vi "canDataSort.vi"() -> ()   [LabVIEW 2023] (continued)
"Min"=0.0, "Max"=65.535, "ScaleFac"=0.001, "ScaleOff"=0.0}, {"1FFFFFFC", "Frame"="PCINPUT\ndatabase", "NameShort"="PCRXMsg7", "StartBit"=48, "NumBits"=16, "Min"=0.0, "Max"=65.535, "ScaleFac"=0.001, "ScaleOff"=0.0}, {"1FFFFFFD", "Frame"="PCOUTPUT\ndatabase", "NameShort"="PCTXMsg1", "StartBit"=0, "NumBits"=16, "Min"=0.0, "Max"=65.535, "ScaleFac"=0.001, "ScaleOff"=0.0}, {"1FFFFFFD", "Frame"="PCOUTPUT\ndatabase", "NameShort"="PCTXMsg3", "StartBit"=16, "NumBits"=16, "Min"=0.0, "Max"=65.535, "ScaleFac"=0.001, "ScaleOff"=0.0}, {"1FFFFFFD", "Frame"="PCOUTPUT\ndatabase", "NameShort"="PCTXMsg5", "StartBit"=32, "NumBits"=16, "Min"=0.0, "Max"=65.535, "ScaleFac"=0.001, "ScaleOff"=0.0}, {"1FFFFFFD", "Frame"="PCOUTPUT\ndatabase", "NameShort"="PCTXMsg7", "StartBit"=48, "NumBits"=16, "Min"=0.0, "Max"=65.535, "ScaleFac"=0.001, "ScaleOff"=0.0}, {"1FFFFFFE", "Frame"="PCRX\ndatabase", "NameShort"="PCRXMsg1", "StartBit"=0, "NumBits"=8, "Min"=0.0, "Max"=255.0, "ScaleFac"=1.0, "ScaleOff"=0.0}, {"1FFFFFFE", "Frame"="PCRX\ndatabase", "NameShort"="PCRXMsg2", "StartBit"=8, "NumBits"=8, "Min"=0.0, "Max"=255.0, "ScaleFac"=1.0, "ScaleOff"=0.0}, {"1FFFFFFE", "Frame"="PCRX\ndatabase", "NameShort"="PCRXMsg3", "StartBit"=16, "NumBits"=8, "Min"=0.0, "Max"=255.0, "ScaleFac"=1.0, "ScaleOff"=0.0}, {"1FFFFFFE", "Frame"="PCRX\ndatabase", "NameShort"="PCRXMsg4", "StartBit"=24, "NumBits"=8, "Min"=0.0, "Max"=255.0, "ScaleFac"=1.0, "ScaleOff"=0.0}, {"1FFFFFFE", "Frame"="PCRX\ndatabase", "NameShort"="PCRXMsg5", "StartBit"=32, "NumBits"=8, "Min"=0.0, "Max"=255.0, "ScaleFac"=1.0, "ScaleOff"=0.0}, {"1FFFFFFE", "Frame"="PCRX\ndatabase", "NameShort"="PCRXMsg6", "StartBit"=40, "NumBits"=8, "Min"=0.0, "Max"=255.0, "ScaleFac"=1.0, "ScaleOff"=0.0}, {"1FFFFFFE", "Frame"="PCRX\ndatabase", "NameShort"="PCRXMsg7", "StartBit"=48, "NumBits"=8, "Min"=0.0, "Max"=255.0, "ScaleFac"=1.0, "ScaleOff"=0.0}, {"1FFFFFFE", "Frame"="PCRX\ndatabase", "NameShort"="PCRXMsg8", "StartBit"=56, "NumBits"=8, "Min"=0.0, "Max"=255.0, "ScaleFac"=1.0, "ScaleOff"=0.0}, {"1FFFFFFF", "Frame"="PCTX\ndatabase", "NameShort"="PCTXMSDI_Gear", "StartBit"=0, "NumBits"=8, "Min"=0.0, "Max"=255.0, "ScaleFac"=1.0, "ScaleOff"=0.0}, {"1FFFFFFF", "Frame"="PCTX\ndatabase", "NameShort"="PCTXMsg2", "StartBit"=8, "NumBits"=8, "Min"=0.0, "Max"=255.0, "ScaleFac"=1.0, "ScaleOff"=0.0}, {"1FFFFFFF", "Frame"="PCTX\ndatabase", "NameShort"="PCTXMsg3", "StartBit"=16, "NumBits"=8, "Min"=0.0, "Max"=255.0, "ScaleFac"=1.0, "ScaleOff"=0.0}, {"1FFFFFFF", "Frame"="PCTX\ndatabase", "NameShort"="PCTXMsg4", "StartBit"=24, "NumBits"=8, "Min"=0.0, "Max"=255.0, "ScaleFac"=1.0, "ScaleOff"=0.0}, {"1FFFFFFF", "Frame"="PCTX\ndatabase", "NameShort"="PCTXMsg5", "StartBit"=32, "NumBits"=8, "Min"=0.0, "Max"=255.0, "ScaleFac"=1.0, "ScaleOff"=0.0}, {"1FFFFFFF", "Frame"="PCTX\ndatabase", "NameShort"="PCTXMsg6", "StartBit"=40, "NumBits"=8, "Min"=0.0, "Max"=255.0, "ScaleFac"=1.0, "ScaleOff"=0.0}, {"1FFFFFFF", "Frame"="PCTX\ndatabase", "NameShort"="PCTXMsg7", "StartBit"=48, "NumBits"=8, "Min"=0.0, "Max"=255.0, "ScaleFac"=1.0, "ScaleOff"=0.0}, {"1FFFFFFF", "Frame"="PCTX\ndatabase", "NameShort"="PCTXMsg8", "StartBit"=56, "NumBits"=8, "Min"=0.0, "Max"=255.0, "ScaleFac"=1.0, "ScaleOff"=0.0}, {"1828A796", "Frame"="SmokeDetector\ndatabase", "NameShort"="SmokeDetectorAlertDeviceAlert", "StartBit"=52, "NumBits"=2, "Min"=0.0, "Max"=1.0, "ScaleFac"=1.0, "ScaleOff"=0.0}, {"1828A796", "Frame"="SmokeDetector\ndatabase", "NameShort"="SmokeDetectorAlertSmokeAlert", "StartBit"=48, "NumBits"=2, "Min"=0.0, "Max"=1.0, "ScaleFac"=1.0, "ScaleOff"=0.0}, {"1828A796", "Frame"="SmokeDetector\ndatabase", "NameShort"="SmokeDetectorAlertTempAlert", "StartBit"=50, "NumBits"=2, "Min"=0.0, "Max"=1.0, "ScaleFac"=1.0, "ScaleOff"=0.0}, {"1828A796", "Frame"="SmokeDetector\ndatabase", "NameShort"="SmokeDetectorLife", "StartBit"=56, "NumBits"=8, "Min"=0.0, "Max"=255.0, "ScaleFac"=1.0, "ScaleOff"=0.0}, {"CF101A7", "Frame"="VCU01toIP\ndatabase", "NameShort"="VCU01BrkPedalDepth", "StartBit"=32, "NumBits"=8, "Min"=0.0, "Max"=100.0, "ScaleFac"=0.4, "ScaleOff"=0.0}, {"CF101A7", "Frame"="VCU01toIP\ndatabase", "NameShort"="VCU01BrkPedalStat", "StartBit"=7, "NumBits"=1, "Min"=0.0, "Max"=1.0, "ScaleFac"=1.0, "ScaleOff"=0.0}, {"CF101A7", "Frame"="VCU01toIP\ndatabase", "NameShort"="VCU01CarSpeed", "StartBit"=16, "NumBits"=16, "Min"=0.0, "Max"=200.0, "ScaleFac"=0.00390625, "ScaleOff"=0.0}, {"CF101A7", "Frame"="VCU01toIP\ndatabase", "NameShort"="VCU01DrivingMode", "StartBit"=0, "NumBits"=2, "Min"=0.0, "Max"=3.0, "ScaleFac"=1.0, "ScaleOff"=0.0}, {"CF101A7", "Frame"="VCU01toIP\ndatabase", "NameShort"="VCU01EESysMalfuctStat", "StartBit"=54, "NumBits"=1, "Min"=0.0, "Max"=1.0, "ScaleFac"=1.0, "ScaleOff"=0.0}, {"CF101A7", "Frame"="VCU01toIP\ndatabase", "NameShort"="VCU01ErrCode", "StartBit"=40, "NumBits"=8, "Min"=0.0, "Max"=255.0, "ScaleFac"=1.0, "ScaleOff"=0.0}, {"CF101A7", "Frame"="VCU01toIP\ndatabase", "NameShort"="VCU01GasPedalDepth", "StartBit"=8, "NumBits"=8, "Min"=0.0, "Max"=100.0, "ScaleFac"=0.4, "ScaleOff"=0.0}, {"CF101A7", "Frame"="VCU01toIP\ndatabase", "NameShort"="VCU01GearStat", "StartBit"=2, "NumBits"=4, "Min"=0.0, "Max"=15.0, "ScaleFac"=1.0, "ScaleOff"=0.0}, {"CF101A7", "Frame"="VCU01toIP\ndatabase", "NameShort"="VCU01HandBrkStat", "StartBit"=6, "NumBits"=1, "Min"=0.0, "Max"=1.0, "ScaleFac"=1.0, "ScaleOff"=0.0}, {"CF101A7", "Frame"="VCU01toIP\ndatabase", "NameShort"="VCU01HillstartAssistIconStat", "StartBit"=50, "NumBits"=1, "Min"=0.0, "Max"=1.0, "ScaleFac"=1.0, "ScaleOff"=0.0}, {"CF101A7", "Frame"="VCU01toIP\ndatabase", "NameShort"="VCU01Life", "StartBit"=56, "NumBits"=8, "Min"=0.0, "Max"=255.0, "ScaleFac"=1.0, "ScaleOff"=0.0}, {"CF101A7", "Frame"="VCU01toIP\ndatabase", "NameShort"="VCU01PowLimitedStat", "StartBit"=49, "NumBits"=1, "Min"=0.0, "Max"=1.0, "ScaleFac"=1.0, "ScaleOff"=0.0}, {"CF101A7", "Frame"="VCU01toIP\ndatabase", "NameShort"="VCU01SysReadyStat", "StartBit"=55, "NumBits"=1, "Min"=0.0, "Max"=1.0, "ScaleFac"=1.0, "ScaleOff"=0.0}, {"CF102A7", "Frame"="VCU02MtrNBMSRelayStat\ndatabase", "NameShort"="VCU02BattOpMode", "StartBit"=38, "NumBits"=2, "Min"=0.0, "Max"=3.0, "ScaleFac"=1.0, "ScaleOff"=0.0}, {"CF102A7", "Frame"="VCU02MtrNBMSRelayStat\ndatabase", "NameShort"="VCU02MtrEnblStat", "StartBit"=37, "NumBits"=1, "Min"=0.0, "Max"=1.0, "ScaleFac"=1.0, "ScaleOff"=0.0}, {"CF102A7", "Frame"="VCU02MtrNBMSRelayStat\ndatabase", "NameShort"="VCU02MtrOpMode", "StartBit"=32, "NumBits"=5, "Min"=0.0, "Max"=31.0, "ScaleFac"=1.0, "ScaleOff"=0.0}, {"CF102A7", "Frame"="VCU02MtrNBMSRelayStat\ndatabase", "NameShort"="VCU02MtrTargetSpeed", "StartBit"=16, "NumBits"=16, "Min"=-12000.0, "Max"=12000.0, "ScaleFac"=1.0, "ScaleOff"=-12000.0}, {"CF102A7", "Frame"="VCU02MtrNBMSRelayStat\ndatabase", "NameShort"="VCU02MtrTargetTorq", "StartBit"=0, "NumBits"=16, "Min"=0.0, "Max"=4095.0, "ScaleFac"=1.0, "ScaleOff"=0.0}, {"CF102A7", "Frame"="VCU02MtrNBMSRelayStat\ndatabase", "NameShort"="VCU02NegRelayStat", "StartBit"=59, "NumBits"=1, "Min"=0.0, "Max"=1.0, "ScaleFac"=1.0, "ScaleOff"=0.0}, {"CF102A7", "Frame"="VCU02MtrNBMSRelayStat\ndatabase", "NameShort"="VCU02PosRelayStat", "StartBit"=58, "NumBits"=1, "Min"=0.0, "Max"=1.0, "ScaleFac"=1.0, "ScaleOff"=0.0}, {"CF102A7", "Frame"="VCU02MtrNBMSRelayStat\ndatabase", "NameShort"="VCU02PrechgRelayStat", "StartBit"=57, "NumBits"=1, "Min"=0.0, "Max"=1.0, "ScaleFac"=1.0, "ScaleOff"=0.0}, {"CF103A7", "Frame"="VCU03VerNFiveInOneRelayStat\ndatabase", "NameShort"="VCU03AirComprNDCDCNEhpsRelayStat", "StartBit"=51, "NumBits"=1, "Min"=0.0, "Max"=1.0, "ScaleFac"=1.0, "ScaleOff"=0.0}, {"CF103A7", "Frame"="VCU03VerNFiveInOneRelayStat\ndatabase", "NameShort"="VCU03AirConRelayStat", "StartBit"=52, "NumBits"=1, "Min"=0.0, "Max"=1.0, "ScaleFac"=1.0, "ScaleOff"=0.0}, {"CF103A7", "Frame"="VCU03VerNFiveInOneRelayStat\ndatabase", "NameShort"="VCU03BattChgRelayCmd", "StartBit"=54, "NumBits"=1, "Min"=0.0, "Max"=1.0, "ScaleFac"=1.0, "ScaleOff"=0.0}, {"CF103A7", "Frame"="VCU03VerNFiveInOneRelayStat\ndatabase", "NameShort"="VCU03BattMainRelayCmd", "StartBit"=55, "NumBits"=1, "Min"=0.0, "Max"=1.0, "ScaleFac"=1.0, "ScaleOff"=0.0}, {"CF103A7", "Frame"="VCU03VerNFiveInOneRelayStat\ndatabase", "NameShort"="VCU03BowtypeChgCmd", "StartBit"=47, "NumBits"=1, "Min"=0.0, "Max"=1.0, "ScaleFac"=1.0, "ScaleOff"=0.0}, {"CF103A7", "Frame"="VCU03VerNFiveInOneRelayStat\ndatabase", "NameShort"="VCU03CompanyCode", "StartBit"=0, "NumBits"=8, "Min"=0.0, "Max"=255.0, "ScaleFac"=1.0, "ScaleOff"=0.0}, {"CF103A7", "Frame"="VCU03VerNFiveInOneRelayStat\ndatabase", "NameShort"="VCU03DefrostRelayStat", "StartBit"=53, "NumBits"=1, "Min"=0.0, "Max"=1.0, "ScaleFac"=1.0, "ScaleOff"=0.0}, {"CF103A7", "Frame"="VCU03VerNFiveInOneRelayStat\ndatabase", "NameShort"="VCU03DriveShaftSpeed", "StartBit"=24, "NumBits"=16, "Min"=-12000.0, "Max"=12000.0, "ScaleFac"=1.0, "ScaleOff"=-12000.0}, {"CF103A7", "Frame"="VCU03VerNFiveInOneRelayStat\ndatabase", "NameShort"="VCU03HVEmergCutoff", "StartBit"=48, "NumBits"=1, "Min"=0.0, "Max"=1.0, "ScaleFac"=1.0, "ScaleOff"=0.0}, {"CF103A7", "Frame"="VCU03VerNFiveInOneRelayStat\ndatabase", "NameShort"="VCU03HwVer", "StartBit"=19, "NumBits"=5, "Min"=0.0, "Max"=31.0, "ScaleFac"=1.0, "ScaleOff"=0.0}, {"CF103A7", "Frame"="VCU03VerNFiveInOneRelayStat\ndatabase", "NameShort"="VCU03Life", "StartBit"=56, "NumBits"=8, "Min"=0.0, "Max"=255.0, "ScaleFac"=1.0, "ScaleOff"=0.0}, {"CF103A7", "Frame"="VCU03VerNFiveInOneRelayStat\ndatabase", "NameShort"="VCU03MtrRelayStat", "StartBit"=50, "NumBits"=1, "Min"=0.0, "Max"=1.0, "ScaleFac"=1.0, "ScaleOff"=0.0}, {"CF103A7", "Frame"="VCU03VerNFiveInOneRelayStat\ndatabase", "NameShort"="VCU03PantographStat", "StartBit"=45, "NumBits"=2, "Min"=0.0, "Max"=3.0, "ScaleFac"=1.0, "ScaleOff"=0.0}, {"CF103A7", "Frame"="VCU03VerNFiveInOneRelayStat\ndatabase", "NameShort"="VCU03PrechgRelayStat", "StartBit"=49, "NumBits"=1, "Min"=0.0, "Max"=1.0, "ScaleFac"=1.0, "ScaleOff"=0.0}, {"CF103A7", "Frame"="VCU03VerNFiveInOneRelayStat\ndatabase", "NameShort"="VCU03SwVer", "StartBit"=8, "NumBits"=11, "Min"=0.0, "Max"=2047.0, "ScaleFac"=1.0, "ScaleOff"=0.0}, {"CF104A7", "Frame"="VCU04toEHPS\ndatabase", "NameShort"="VCU04EHPSAssignRPM", "StartBit"=8, "NumBits"=16, "Min"=0.0, "Max"=5000.0, "ScaleFac"=0.125, "ScaleOff"=0.0}, {"CF104A7", "Frame"="VCU04toEHPS\ndatabase", "NameShort"="VCU04EHPSEnbl1", "StartBit"=0, "NumBits"=2, "Min"=0.0, "Max"=3.0, "ScaleFac"=1.0, "ScaleOff"=0.0}, {"CF104A7", "Frame"="VCU04toEHPS\ndatabase", "NameShort"="VCU04EHPSEnbl2", "StartBit"=2, "NumBits"=2, "Min"=0.0, "Max"=3.0, "ScaleFac"=1.0, "ScaleOff"=0.0}, {"CF104A7", "Frame"="VCU04toEHPS\ndatabase", "NameShort"="VCU04EHPSLVEnbl", "StartBit"=24, "NumBits"=2, "Min"=0.0, "Max"=3.0, "ScaleFac"=1.0, "ScaleOff"=0.0}, {"CF104A7", "Frame"="VCU04toEHPS\ndatabase", "NameShort"="VCU04EHPSLife", "StartBit"=56, "NumBits"=8, "Min"=0.0, "Max"=255.0, "ScaleFac"=1.0, "ScaleOff"=0.0}, {"C3C4D4A", "Frame"="VCU05toAirCon\ndatabase", "NameShort"="VCU05AirConEnbl", "StartBit"=6, "NumBits"=1, "Min"=0.0, "Max"=1.0, "ScaleFac"=1.0, "ScaleOff"=0.0}, {"C3C4D4A", "Frame"="VCU05toAirCon\ndatabase", "NameShort"="VCU05AirConLife", "StartBit"=56, "NumBits"=8, "Min"=0.0, "Max"=255.0, "ScaleFac"=1.0, "ScaleOff"=0.0}, {"C3C4D4A", "Frame"="VCU05toAirCon\ndatabase", "NameShort"="VCU05AirConRead24VVolt", "StartBit"=32, "NumBits"=8, "Min"=0.0, "Max"=40.0, "ScaleFac"=1.0, "ScaleOff"=0.0}, {"C3C4D4A", "Frame"="VCU05toAirCon\ndatabase", "NameShort"="VCU05AirConReadSOC", "StartBit"=48, "NumBits"=16, "Min"=0.0, "Max"=100.0, "ScaleFac"=0.4, "ScaleOff"=0.0}, {"C3C4D4A", "Frame"="VCU05toAirCon\ndatabase", "NameShort"="VCU05AirConResetCmd", "StartBit"=0, "NumBits"=1, "Min"=0.0, "Max"=1.0, "ScaleFac"=1.0, "ScaleOff"=0.0}, {"C3C4D4A", "Frame"="VCU05toAirCon\ndatabase", "NameShort"="VCU05AirConRsvdUsing1", "StartBit"=31, "NumBits"=1, "Min"=0.0, "Max"=1.0, "ScaleFac"=1.0, "ScaleOff"=0.0}, {"CF105A7", "Frame"="VCU06toDCDC\ndatabase", "NameShort"="VCU06DCDCEnblCmd", "StartBit"=24, "NumBits"=8, "Min"=0.0, "Max"=255.0, "ScaleFac"=1.0, "ScaleOff"=0.0}, {"CF105A7", "Frame"="VCU06toDCDC\ndatabase", "NameShort"="VCU06DCDCEnblReqOutOf24V", "StartBit"=16, "NumBits"=8, "Min"=0.0, "Max"=255.0, "ScaleFac"=1.0, "ScaleOff"=0.0}, {"CF105A7", "Frame"="VCU06toDCDC\ndatabase", "NameShort"="VCU06DCDCLife", "StartBit"=56, "NumBits"=8, "Min"=0.0, "Max"=255.0, "ScaleFac"=1.0, "ScaleOff"=0.0}, {"CF105A7", "Frame"="VCU06toDCDC\ndatabase", "NameShort"="VCU06DCDCMinHVReq", "StartBit"=0, "NumBits"=16, "Min"=0.0, "Max"=6553.5, "ScaleFac"=0.1, "ScaleOff"=0.0}, {"18F106A7", "Frame"="VCU07toFiveInOneRelay\ndatabase", "NameShort"="VCU07FiveInOneAirComprRelayCmd", "StartBit"=3, "NumBits"=1, "Min"=0.0, "Max"=1.0, "ScaleFac"=1.0, "ScaleOff"=0.0}, {"18F106A7", "Frame"="VCU07toFiveInOneRelay\ndatabase", "NameShort"="VCU07FiveInOneAirConRelayCmd", "StartBit"=2, "NumBits"=1, "Min"=0.0, "Max"=1.0, "ScaleFac"=1.0, "ScaleOff"=0.0}, {"18F106A7", "Frame"="VCU07toFiveInOneRelay\ndatabase", "NameShort"="VCU07FiveInOneBrkResistRelayCmd", "StartBit"=11, "NumBits"=1, "Min"=0.0, "Max"=1.0, "ScaleFac"=1.0, "ScaleOff"=0.0}, {"18F106A7", "Frame"="VCU07toFiveInOneRelay\ndatabase", "NameShort"="VCU07FiveInOneDCDCRelayCmd", "StartBit"=5, "NumBits"=1, "Min"=0.0, "Max"=1.0, "ScaleFac"=1.0, "ScaleOff"=0.0}, {"18F106A7", "Frame"="VCU07toFiveInOneRelay\ndatabase", "NameShort"="VCU07FiveInOneDefrostRelayCmd", "StartBit"=1, "NumBits"=1, "Min"=0.0, "Max"=1.0, "ScaleFac"=1.0, "ScaleOff"=0.0}, {"18F106A7", "Frame"="VCU07toFiveInOneRelay\ndatabase", "NameShort"="VCU07FiveInOneEHPSRelayCmd", "StartBit"=4, "NumBits"=1, "Min"=0.0, "Max"=1.0, "ScaleFac"=1.0, "ScaleOff"=0.0}, {"18F106A7", "Frame"="VCU07toFiveInOneRelay\ndatabase", "NameShort"="VCU07FiveInOneHeatRelayCmd", "StartBit"=0, "NumBits"=1, "Min"=0.0, "Max"=1.0, "ScaleFac"=1.0, "ScaleOff"=0.0}, {"18F106A7", "Frame"="VCU07toFiveInOneRelay\ndatabase", "NameShort"="VCU07FiveInOneLife", "StartBit"=56, "NumBits"=8, "Min"=0.0, "Max"=255.0, "ScaleFac"=1.0, "ScaleOff"=0.0}, {"18F106A7", "Frame"="VCU07toFiveInOneRelay\ndatabase", "NameShort"="VCU07FiveInOneMtrRelayCmd", "StartBit"=6, "NumBits"=1, "Min"=0.0, "Max"=1.0, "ScaleFac"=1.0, "ScaleOff"=0.0}, {"18F106A7", "Frame"="VCU07toFiveInOneRelay\ndatabase", "NameShort"="VCU07FiveInOnePrechgRelayCmd", "StartBit"=7, "NumBits"=1, "Min"=0.0, "Max"=1.0, "ScaleFac"=1.0, "ScaleOff"=0.0}, {"18F108A7", "Frame"="VCU08toAirCompr1\ndatabase", "NameShort"="VCU08AirComprAssignRPM", "StartBit"=8, "NumBits"=16, "Min"=0.0, "Max"=5000.0, "ScaleFac"=0.125, "ScaleOff"=0.0}, {"18F108A7", "Frame"="VCU08toAirCompr1\ndatabase", "NameShort"="VCU08AirComprEnbl1", "StartBit"=0, "NumBits"=2, "Min"=0.0, "Max"=3.0, "ScaleFac"=1.0, "ScaleOff"=0.0}, {"18F108A7", "Frame"="VCU08toAirCompr1\ndatabase", "NameShort"="VCU08AirComprEnbl2", "StartBit"=2, "NumBits"=2, "Min"=0.0, "Max"=3.0, "ScaleFac"=1.0, "ScaleOff"=0.0}, {"18F108A7", "Frame"="VCU08toAirCompr1\ndatabase", "NameShort"="VCU08AirComprLife", "StartBit"=56, "NumBits"=8, "Min"=0.0, "Max"=255.0, "ScaleFac"=1.0, "ScaleOff"=0.0}, {"18F109A7", "Frame"="VCU09toAirCompr2\ndatabase", "NameShort"="VCU09AirComprAssignRPM", "StartBit"=8, "NumBits"=16, "Min"=0.0, "Max"=5000.0, "ScaleFac"=0.125, "ScaleOff"=0.0}, {"18F109A7", "Frame"="VCU09toAirCompr2\ndatabase", "NameShort"="VCU09AirComprEnbl1", "StartBit"=0, "NumBits"=2, "Min"=0.0, "Max"=3.0, "ScaleFac"=1.0, "ScaleOff"=0.0}, {"18F109A7", "Frame"="VCU09toAirCompr2\ndatabase", "NameShort"="VCU09AirComprEnbl2", "StartBit"=2, "NumBits"=2, "Min"=0.0, "Max"=3.0, "ScaleFac"=1.0, "ScaleOff"=0.0}, {"18F109A7", "Frame"="VCU09toAirCompr2\ndatabase", "NameShort"="VCU09AirComprLife", "StartBit"=56, "NumBits"=8, "Min"=0.0, "Max"=255.0, "ScaleFac"=1.0, "ScaleOff"=0.0}, {"CF109A7", "Frame"="VCU10toBrkResistNBMS\ndatabase", "NameShort"="VCU10BattMainRelayCmd", "StartBit"=55, "NumBits"=1, "Min"=0.0, "Max"=1.0, "ScaleFac"=1.0, "ScaleOff"=0.0}, {"CF109A7", "Frame"="VCU10toBrkResistNBMS\ndatabase", "NameShort"="VCU10BattMaxChgPowAllowed", "StartBit"=16, "NumBits"=16, "Min"=0.0, "Max"=500.0, "ScaleFac"=1.0, "ScaleOff"=0.0}, {"CF109A7", "Frame"="VCU10toBrkResistNBMS\ndatabase", "NameShort"="VCU10BrkResistNBMSLife", "StartBit"=56, "NumBits"=8, "Min"=0.0, "Max"=255.0, "ScaleFac"=1.0, "ScaleOff"=0.0}, {"CF109A7", "Frame"="VCU10toBrkResistNBMS\ndatabase", "NameShort"="VCU10BrkResistPowCmd", "StartBit"=47, "NumBits"=1, "Min"=0.0, "Max"=1.0, "ScaleFac"=1.0, "ScaleOff"=0.0}, {"CF109A7", "Frame"="VCU10toBrkResistNBMS\ndatabase", "NameShort"="VCU10BrkResistPowConsumpReq", "StartBit"=0, "NumBits"=16, "Min"=0.0, "Max"=500.0, "ScaleFac"=1.0, "ScaleOff"=0.0}, {"CF109A7", "Frame"="VCU10toBrkResistNBMS\ndatabase", "NameShort"="VCU10BrkResistorPowONOFFCmd", "StartBit"=46, "NumBits"=1, "Min"=0.0, "Max"=1.0, "ScaleFac"=1.0, "ScaleOff"=0.0}, {"18F10BA7", "Frame"="VCU11EVEff\ndatabase", "NameShort"="VCU11AvgPowConsump", "StartBit"=16, "NumBits"=16, "Min"=0.0, "Max"=5000.0, "ScaleFac"=0.1, "ScaleOff"=0.0}, {"18F10BA7", "Frame"="VCU11EVEff\ndatabase", "NameShort"="VCU11IPLife", "StartBit"=56, "NumBits"=8, "Min"=0.0, "Max"=255.0, "ScaleFac"=1.0, "ScaleOff"=0.0}, {"18F10BA7", "Frame"="VCU11EVEff\ndatabase", "NameShort"="VCU11InstantPowConsump", "StartBit"=0, "NumBits"=16, "Min"=0.0, "Max"=5000.0, "ScaleFac"=0.1, "ScaleOff"=0.0}, {"18F10BA7", "Frame"="VCU11EVEff\ndatabase", "NameShort"="VCU11RemainMileage", "StartBit"=32, "NumBits"=16, "Min"=0.0, "Max"=5000.0, "ScaleFac"=1.0, "ScaleOff"=0.0}, {"18FB01A7", "Frame"="VCU12AVAS\ndatabase", "NameShort"="VCU12AVASAcousticVehicleAlertSys", "StartBit"=12, "NumBits"=4, "Min"=0.0, "Max"=15.0, "ScaleFac"=1.0, "ScaleOff"=0.0}, {"18FEC1A7", "Frame"="VCU13Mileage\ndatabase", "NameShort"="VCU13MileageTotalOdometer", "StartBit"=0, "NumBits"=32, "Min"=0.0, "Max"=21055406.0, "ScaleFac"=0.005, "ScaleOff"=0.0}, {"18FEF117", "Frame"="VCU14CCVS\ndatabase", "NameShort"="VCU14CCVSBrkSwitch", "StartBit"=28, "NumBits"=2, "Min"=0.0, "Max"=3.0, "ScaleFac"=1.0, "ScaleOff"=0.0}, {"18FEF117", "Frame"="VCU14CCVS\ndatabase", "NameShort"="VCU14CCVSClutchSwitch", "StartBit"=30, "NumBits"=2, "Min"=0.0, "Max"=3.0, "ScaleFac"=1.0, "ScaleOff"=0.0}, {"18FEF117", "Frame"="VCU14CCVS\ndatabase", "NameShort"="VCU14CCVSCruiseCtrlAccSwitch", "StartBit"=38, "NumBits"=2, "Min"=0.0, "Max"=3.0, "ScaleFac"=1.0, "ScaleOff"=0.0}, {"18FEF117", "Frame"="VCU14CCVS\ndatabase", "NameShort"="VCU14CCVSCruiseCtrlActive", "StartBit"=24, "NumBits"=2, "Min"=0.0, "Max"=3.0, "ScaleFac"=1.0, "ScaleOff"=0.0}, {"18FEF117", "Frame"="VCU14CCVS\ndatabase", "NameShort"="VCU14CCVSCruiseCtrlCoastSwitch", "StartBit"=34, "NumBits"=2, "Min"=0.0, "Max"=3.0, "ScaleFac"=1.0, "ScaleOff"=0.0}, {"18FEF117", "Frame"="VCU14CCVS\ndatabase", "NameShort"="VCU14CCVSCruiseCtrlEnblSwitch", "StartBit"=26, "NumBits"=2, "Min"=0.0, "Max"=3.0, "ScaleFac"=1.0, "ScaleOff"=0.0}, {"18FEF117", "Frame"="VCU14CCVS\ndatabase", "NameShort"="VCU14CCVSCruiseCtrlPauseSwitch", "StartBit"=4, "NumBits"=2, "Min"=0.0, "Max"=3.0, "ScaleFac"=1.0, "ScaleOff"=0.0}, {"18FEF117", "Frame"="VCU14CCVS\ndatabase", "NameShort"="VCU14CCVSCruiseCtrlResumeSwitch", "StartBit"=36, "NumBits"=2, "Min"=0.0, "Max"=3.0, "ScaleFac"=1.0, "ScaleOff"=0.0}, {"18FEF117", "Frame"="VCU14CCVS\ndatabase", "NameShort"="VCU14CCVSCruiseCtrlSetSpeed", "StartBit"=40, "NumBits"=8, "Min"=0.0, "Max"=255.0, "ScaleFac"=1.0, "ScaleOff"=0.0}, {"18FEF117", "Frame"="VCU14CCVS\ndatabase", "NameShort"="VCU14CCVSCruiseCtrlSetSwitch", "StartBit"=32, "NumBits"=2, "Min"=0.0, "Max"=3.0, "ScaleFac"=1.0, "ScaleOff"=0.0}, {"18FEF117", "Frame"="VCU14CCVS\ndatabase", "NameShort"="VCU14CCVSCruiseCtrlState", "StartBit"=53, "NumBits"=3, "Min"=0.0, "Max"=7.0, "ScaleFac"=1.0, "ScaleOff"=0.0}, {"18FEF117", "Frame"="VCU14CCVS\ndatabase", "NameShort"="VCU14CCVSEngIdleDecrementSwitch", "StartBit"=58, "NumBits"=2, "Min"=0.0, "Max"=3.0, "ScaleFac"=1.0, "ScaleOff"=0.0}, {"18FEF117", "Frame"="VCU14CCVS\ndatabase", "NameShort"="VCU14CCVSEngIdleIncrementSwitch", "StartBit"=56, "NumBits"=2, "Min"=0.0, "Max"=3.0, "ScaleFac"=1.0, "ScaleOff"=0.0}, {"18FEF117", "Frame"="VCU14CCVS\ndatabase", "NameShort"="VCU14CCVSEngShutdownOvrSwitch", "StartBit"=62, "NumBits"=2, "Min"=0.0, "Max"=3.0, "ScaleFac"=1.0, "ScaleOff"=0.0}, {"18FEF117", "Frame"="VCU14CCVS\ndatabase", "NameShort"="VCU14CCVSEngTestModeSwitch", "StartBit"=60, "NumBits"=2, "Min"=0.0, "Max"=3.0, "ScaleFac"=1.0, "ScaleOff"=0.0}, {"18FEF117", "Frame"="VCU14CCVS\ndatabase", "NameShort"="VCU14CCVSPTOGovernorState", "StartBit"=48, "NumBits"=5, "Min"=0.0, "Max"=31.0, "ScaleFac"=1.0, "ScaleOff"=0.0}, {"18FEF117", "Frame"="VCU14CCVS\ndatabase", "NameShort"="VCU14CCVSParkBrkReleaseInhibitRq", "StartBit"=6, "NumBits"=2, "Min"=0.0, "Max"=3.0, "ScaleFac"=1.0, "ScaleOff"=0.0}, {"18FEF117", "Frame"="VCU14CCVS\ndatabase", "NameShort"="VCU14CCVSParkingBrkSwitch", "StartBit"=2, "NumBits"=2, "Min"=0.0, "Max"=3.0, "ScaleFac"=1.0, "ScaleOff"=0.0}, {"18FEF117", "Frame"="VCU14CCVS\ndatabase", "NameShort"="VCU14CCVSTwoSpeedAxleSwitch", "StartBit"=0, "NumBits"=2, "Min"=0.0, "Max"=3.0, "ScaleFac"=1.0, "ScaleOff"=0.0}, {"18FEF117", "Frame"="VCU14CCVS\ndatabase", "NameShort"="VCU14CCVSWheelBasedVehicleSpeed", "StartBit"=8, "NumBits"=16, "Min"=0.0, "Max"=250.996, "ScaleFac"=0.00390625, "ScaleOff"=0.0}, {"18F10CA7", "Frame"="VCU15VIN\ndatabase", "NameShort"="VCU15VINPkgNum", "StartBit"=0, "NumBits"=8, "Min"=0.0, "Max"=255.0, "ScaleFac"=1.0, "ScaleOff"=0.0}, {"18F10CA7", "Frame"="VCU15VIN\ndatabase", "NameShort"="VCU15VINcode0", "StartBit"=8, "NumBits"=8, "Min"=0.0, "Max"=255.0, "ScaleFac"=1.0, "ScaleOff"=0.0}, {"18F10CA7", "Frame"="VCU15VIN\ndatabase", "NameShort"="VCU15VINcode1", "StartBit"=16, "NumBits"=8, "Min"=0.0, "Max"=255.0, "ScaleFac"=1.0, "ScaleOff"=0.0}, {"18F10CA7", "Frame"="VCU15VIN\ndatabase", "NameShort"="VCU15VINcode2", "StartBit"=24, "NumBits"=8, "Min"=0.0, "Max"=255.0, "ScaleFac"=1.0, "ScaleOff"=0.0}, {"18F10CA7", "Frame"="VCU15VIN\ndatabase", "NameShort"="VCU15VINcode3", "StartBit"=32, "NumBits"=8, "Min"=0.0, "Max"=255.0, "ScaleFac"=1.0, "ScaleOff"=0.0}, {"18F10CA7", "Frame"="VCU15VIN\ndatabase", "NameShort"="VCU15VINcode4", "StartBit"=40, "NumBits"=8, "Min"=0.0, "Max"=255.0, "ScaleFac"=1.0, "ScaleOff"=0.0}, {"18F10CA7", "Frame"="VCU15VIN\ndatabase", "NameShort"="VCU15VINcode5", "StartBit"=48, "NumBits"=8, "Min"=0.0, "Max"=255.0, "ScaleFac"=1.0, "ScaleOff"=0.0}, {"18F10CA7", "Frame"="VCU15VIN\ndatabase", "NameShort"="VCU15VINcode6", "StartBit"=56, "NumBits"=8, "Min"=0.0, "Max"=255.0, "ScaleFac"=1.0, "ScaleOff"=0.0}, {"CF101D0", "Frame"="VCUtoINVT\ndatabase", "NameShort"="VCUtoINVTACHVPowReq", "StartBit"=24, "NumBits"=2, "Min"=0.0, "Max"=3.0, "ScaleFac"=1.0, "ScaleOff"=0.0}, {"CF101D0", "Frame"="VCUtoINVT\ndatabase", "NameShort"="VCUtoINVTLife", "StartBit"=56, "NumBits"=8, "Min"=0.0, "Max"=255.0, "ScaleFac"=1.0, "ScaleOff"=0.0}, {"CF101D0", "Frame"="VCUtoINVT\ndatabase", "NameShort"="VCUtoINVTMCUHVPowReq", "StartBit"=8, "NumBits"=2, "Min"=0.0, "Max"=3.0, "ScaleFac"=1.0, "ScaleOff"=0.0}, {"CF103D0", "Frame"="VCUtoINVT2\ndatabase", "NameShort"="VCUtoINVT2DCDCEnbl", "StartBit"=4, "NumBits"=2, "Min"=0.0, "Max"=1.0, "ScaleFac"=1.0, "ScaleOff"=0.0}, {"CF103D0", "Frame"="VCUtoINVT2\ndatabase", "NameShort"="VCUtoINVT2DCDCOUTVolt", "StartBit"=8, "NumBits"=16, "Min"=0.0, "Max"=6553.5, "ScaleFac"=0.1, "ScaleOff"=0.0}, {"CF103D0", "Frame"="VCUtoINVT2\ndatabase", "NameShort"="VCUtoINVT2EACEnbl", "StartBit"=2, "NumBits"=2, "Min"=0.0, "Max"=1.0, "ScaleFac"=1.0, "ScaleOff"=0.0}, {"CF103D0", "Frame"="VCUtoINVT2\ndatabase", "NameShort"="VCUtoINVT2EACmode", "StartBit"=7, "NumBits"=1, "Min"=0.0, "Max"=1.0, "ScaleFac"=1.0, "ScaleOff"=0.0}, {"CF103D0", "Frame"="VCUtoINVT2\ndatabase", "NameShort"="VCUtoINVT2EACrpm", "StartBit"=40, "NumBits"=16, "Min"=-5000.0, "Max"=5000.0, "ScaleFac"=0.5, "ScaleOff"=-5000.0}, {"CF103D0", "Frame"="VCUtoINVT2\ndatabase", "NameShort"="VCUtoINVT2EHPSEnbl", "StartBit"=0, "NumBits"=2, "Min"=0.0, "Max"=1.0, "ScaleFac"=1.0, "ScaleOff"=0.0}, {"CF103D0", "Frame"="VCUtoINVT2\ndatabase", "NameShort"="VCUtoINVT2EHPSmode", "StartBit"=6, "NumBits"=1, "Min"=0.0, "Max"=1.0, "ScaleFac"=1.0, "ScaleOff"=0.0}, {"CF103D0", "Frame"="VCUtoINVT2\ndatabase", "NameShort"="VCUtoINVT2EHPSrpm", "StartBit"=24, "NumBits"=16, "Min"=-5000.0, "Max"=5000.0, "ScaleFac"=0.5, "ScaleOff"=-5000.0}, {"CF103D0", "Frame"="VCUtoINVT2\ndatabase", "NameShort"="VCUtoINVT2Life", "StartBit"=56, "NumBits"=8, "Min"=0.0, "Max"=255.0, "ScaleFac"=1.0, "ScaleOff"=0.0}]
  # "VCU1:ID=0x0CF101A7"
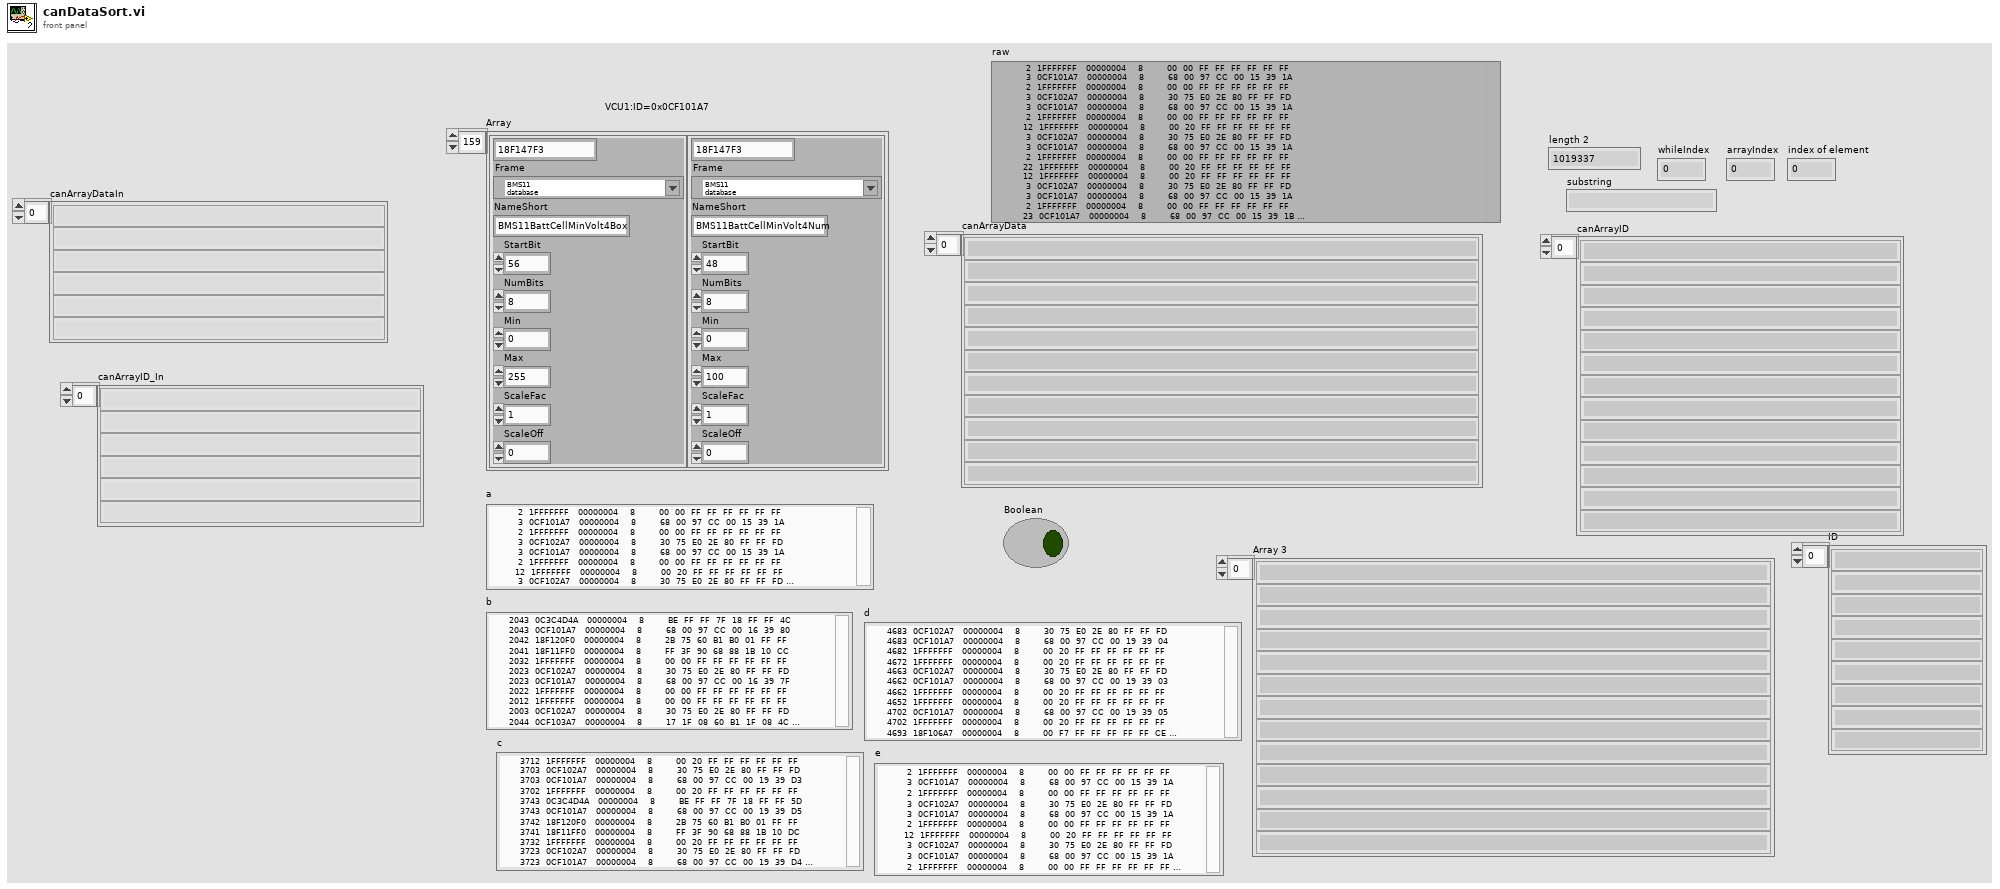
[diagram p1: front panel]
types:
  T1 = cluster{string, "Frame":refnum<k21>, "NameShort":string, "StartBit":u32, "NumBits":u32, "Min":dbl, "Max":dbl, "ScaleFac":dbl, "ScaleOff":dbl}[]
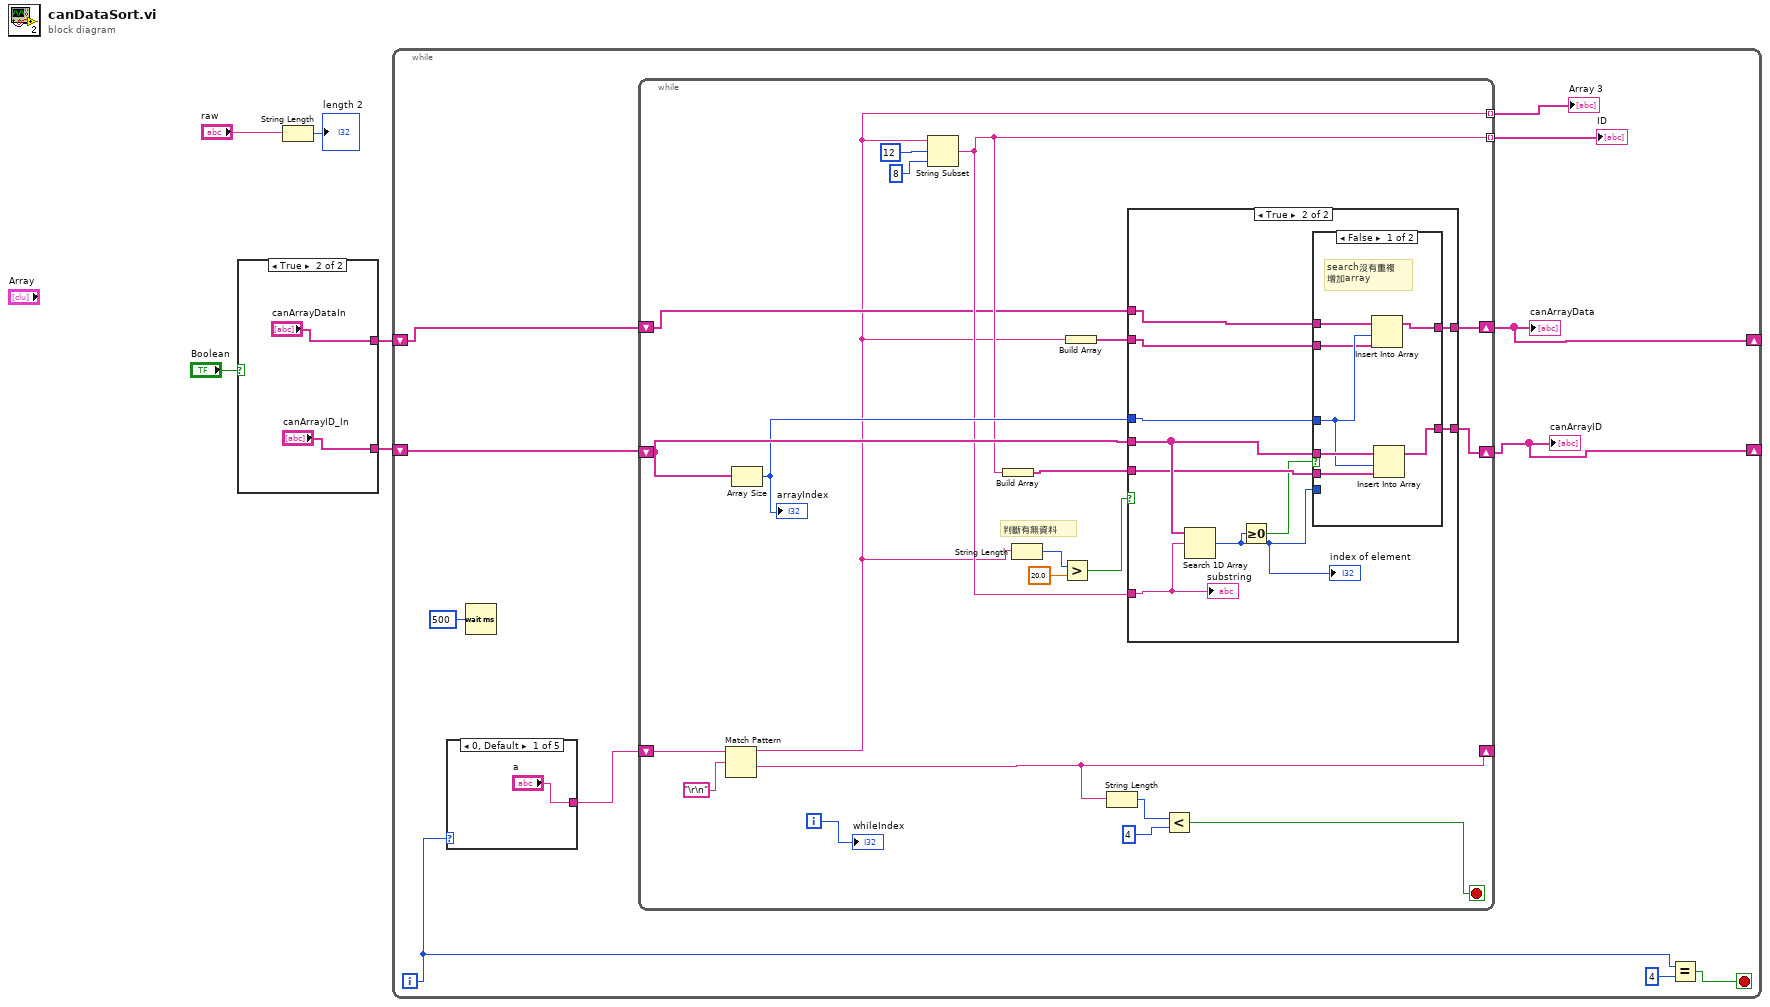
[diagram p0: block diagram]
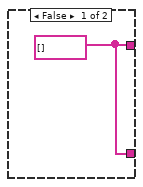
[diagram p2: hidden frame]
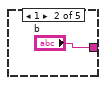
[diagram p3: hidden frame]
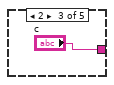
[diagram p4: hidden frame]
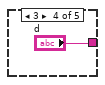
[diagram p5: hidden frame]
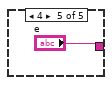
[diagram p6: hidden frame]
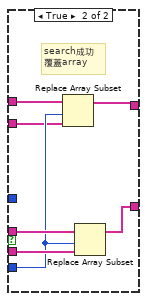
[diagram p8: hidden frame]
diagram:
  n1 = case shown="True" "Boolean" {
    tunnel: [w6 "canArrayDataIn"] -> w3
    tunnel: [w6 "canArrayID_In"] -> w2
    frame False {
      w6 = string[] [] ("appended array")
    }
    frame True {
    }
  }
  n2 = String Length(string="raw") -> (length=→"length 2":i32)
  n3 = while {
    shift-right: [w14] -> _
    shift-left: w2 -> [w13]
    shift-right: [w11] -> _
    shift-left: w3 -> [w12]
    i -> [w10]
    stop <- w18 stop-if-true
    n4 = case shown="0, Default" w10 {
      tunnel: ["a" "b" "c" "d" "e"] -> w19
      frame 0, Default {
      }
      frame 1 {
      }
      frame 2 {
      }
      frame 3 {
      }
      frame 4 {
      }
    }
    n5 = Wait (ms)(milliseconds to wait=u32 500) -> ()  [unwired: 1 out]
    n6 = while {
      shift-right: [w44] -> _
      shift-left: w19 -> [w40]
      tunnel: [w28] -> w16 mode=indexing
      tunnel: [w32] -> w15 mode=indexing
      shift-right: [w35] -> w14
      shift-left: w13 -> [w36]
      shift-right: [w30] -> w11
      shift-left: w12 -> [w31]
      i -> [w34]
      stop <- w41 stop-if-true
      # "判斷有無資料"
      n7 = Match Pattern(string=w40, regular expression="\r\n") -> (before substring=w28:string, after substring=w44:string)  [unwired: 1 in, 2 out]
      n8 = Array Size(array=w36) -> (size(s)=w33:i32)
      "arrayIndex" <- w33
      n9 = String Subset(string=w28, offset (0)=12, length (rest)=8 ("offset (0)")) -> (substring=w32:string)
      n10 = Build Array(w32) -> (w37:string[])
      n11 = String Length(string=w28) -> (length=w26:i32)
      n12 = Greater?(x=w26, y=20.0) -> (0:w25:bool)
      n13 = Build Array(w28) -> (w29:string[])
      n14 = String Length(string=w44) -> (length=w43:i32)
      n15 = case shown="True" w25 {
        tunnel: w37 -> [_ w55]
        tunnel: w36 -> [w47 w56]
        tunnel: [w47 w57] -> w35
        tunnel: w33 -> [_ w51]
        tunnel: w32 -> [_ w54]
        tunnel: w31 -> [w46 w48]
        tunnel: [w46 w50] -> w30
        tunnel: w29 -> [_ w49]
        frame False {
        }
        frame True {
          n16 = Search 1D Array(1D array=w56, element=w54) -> (index of element=w52:i32)  [unwired: 1 in]
          "index of element" <- w52
          n17 = Greater Or Equal To 0?(x=w52) -> (x >= 0?=w53:bool)
          n18 = case shown="False" w53 {
            tunnel: [w64 w69] -> w57
            tunnel: w56 -> [w63 w71]
            tunnel: w55 -> [w62 w70]
            tunnel: w52 -> [_ w66]
            tunnel: w51 -> [w60 _]
            tunnel: [w61 w68] -> w50
            tunnel: w49 -> [w59 w65]
            tunnel: w48 -> [w58 w67]
            frame False {
              # "search沒有重複\n增加array"
              n19 = Insert Into Array(array=w58, index=w60, new element=w59) -> (w61:string[])
              n20 = Insert Into Array(array=w63, index=w60, new element=w62) -> (w64:string[])
            }
            frame True {
              # "search成功\n覆蓋array"
              n21 = Replace Array Subset(array=w67, new element=w65, index=w66) -> (w68:string[])
              n22 = Replace Array Subset(array=w71, new element=w70, index=w66) -> (w69:string[])
            }
          }
          "substring" <- w54
        }
      }
      n23 = Less?(x=w43, y=4) -> (x < y?=w41:bool)
      "whileIndex" <- w34
    }
    "Array 3" <- w16
    "ID" <- w15
    "canArrayID" <- w14
    "canArrayData" <- w11
    n24 = Equal?(x=w10, y=4) -> (x = y?=w18:bool)
  }
